vi "initialise.vi"(8 "error in (no error)":errorcluster, 10 "computer name":string) -> (0 "error out":errorcluster, 3 "FileNeologist out":refnum<class "FileNeologist.lvclass">)   [LabVIEW 2009, in "Tools.lvlib" / "Filing.lvlib" / "FileNeologist.lvclass"]
doc: "FileNeologist Initialise.\n\nThe File Neologist is responsible for creating new files, and naming/renaming files."
uses:
  FileNeologist.lvclass
  FileNeologist.lvclass/FileNeologist.ctl
  FileSystem/FileSystem.lvclass
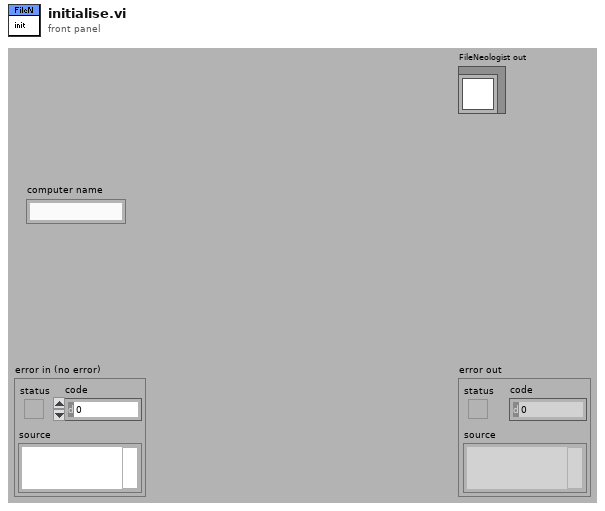
[diagram p1: front panel]
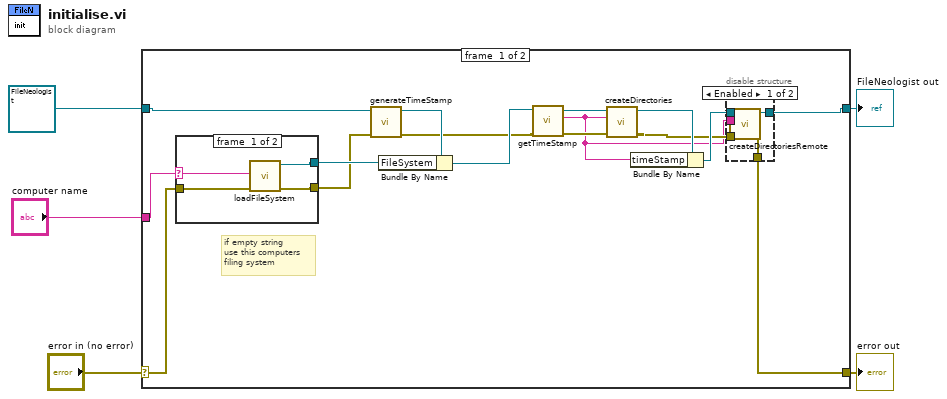
[diagram p0: block diagram]
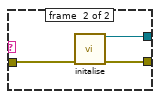
[diagram p3: hidden frame]
diagram:
  n1 = case shown="No Error" "error in (no error)" {
    selector: "error in (no error)" -> [w21 w37]
    tunnel: [w8 w37] -> w4
    tunnel: [w7 w36] -> w3
    tunnel: refnum<class "FileNeologist.lvclass"> refnum ("Tools.lvlib:Filing.lvlib:FileNeologist.lvclass") -> [w14 w36]
    tunnel: "computer name" -> [w15 _]
    frame #0 {
      # "if empty string\nuse this computers\nfiling system"
      n2 = case shown="\"\"" w15 {
        selector: w15 -> [w32 _]
        tunnel: w21 -> [w29 w35]
        tunnel: [w31 w34] -> w20
        tunnel: [w30 w33] -> w11
        frame #0 {
          n3 = call "loadFileSystem.vi"("error in (no error)"=w29, "computer name"=w32) -> ("error out"=w30:errorcluster, "FileSystem out"=w31:refnum<class "FileSystem.lvclass">)  [unwired: 8 in]
        }
        frame #1 {
          n4 = call "initalise.vi"("error in (no error)"=w35) -> ("error out"=w33:errorcluster, "FileSystem out"=w34:refnum<class "FileSystem.lvclass">)  [unwired: 9 in]
        }
      }
      n5 = call "generateTimeStamp.vi"("error in (no error)"=w11, "FileNeologist in"=w14) -> ("error out"=w12:errorcluster, "FileNeologist out"=w13:refnum<class "FileNeologist.lvclass">)  [unwired: 8 in]
      n6 = Bundle By Name(cluster=w13, "FileSystem"=w20) -> (w19:refnum<class "FileNeologist.lvclass">)
      n7 = call "getTimeStamp.vi"("error in (no error)"=w12, "FileNeologist in"=w19) -> ("error out"=w17:errorcluster, "TimeStamp"=w6:string, "FileNeologist out"=w18:refnum<class "FileNeologist.lvclass">)  [unwired: 7 in]
      n8 = call "createDirectories.vi"("error in (no error)"=w17, "TimeStamp"=w6, "FileNeologist in"=w18) -> ("error out"=w9:errorcluster, "FileNeologist out"=w16:refnum<class "FileNeologist.lvclass">)  [unwired: 7 in]
      n9 = Bundle By Name(cluster=w16, "timeStamp"=w6) -> (w10:refnum<class "FileNeologist.lvclass">)
      n10 = disable-structure shown="Enabled" {
        disable-tunnel: w10 -> [w26 w28]
        disable-tunnel: w9 -> [w25 w27]
        disable-tunnel: [w24 w27] -> w8
        disable-tunnel: [w23 w28] -> w7
        disable-tunnel: w6 -> [w22 _]
        frame #0 {
          n11 = call "createDirectoriesRemote.vi"("error in (no error)"=w25, "TimeStamp"=w22, "FileNeologist in"=w26) -> ("error out"=w24:errorcluster, "FileNeologist out"=w23:refnum<class "FileNeologist.lvclass">)  [unwired: 7 in]
        }
        frame #1 {
        }
      }
    }
    frame #1 {
    }
  }
  "error out" <- w4
  "FileNeologist out" <- w3
